vi "Keithley 24XX Output List and Acquire.vi"() -> ()   [LabVIEW 2022 SP3]
doc: "Outputs a sequence of voltages based on a list and takes readings at each point."
uses:
  Keithley 24XX.lvlib
  Initialize Folder/D/Download/Keithley 24XX/Public/Data/Read (Multiple Points).vi
panel:
  in  "Source Mode  (0: Voltage)":u16(ring) items=["Voltage", "Current"]
  in  "Output List":dbl[](array[numeric])=[0.1, 0.2, 0.3]
  in  "VISA resource name":refnum<visa-resource-name>
  in  "Serial Configuration":T1={"Baud Rate"=9600, "Parity"=0, "Data Bits"=8, "Stop Bits"=10, "Flow Control"=0} {"Flow Control" items=["None", "XON/XOFF", "RTS/CTS", "XON/XOFF & RTS/CTS", "DTR/DSR", "XON/XOFF & DTR/DSR"]; "Stop Bits" items=["1.0"=10, "1.5"=15, "2.0"=20]; "Data Bits" items=["7"=7, "8"=8]; "Parity" items=["None", "Odd", "Even", "Mark", "Space"]; "Baud Rate" items=["300"=300, "600"=600, "1200"=1200, "2400"=2400, "4800"=4800, "9600"=9600, "19200"=19200]}
  out "Waveform Graph":sgl[][](graph)
  in  "Timeout (10000 ms)":i32=10000 format="%#.6g"
  in  "Compliance  Level (0.1)":dbl=0.1
  # "(c) 2006 - 2015 National Instruments.  ALL RIGHTS RESERVED."
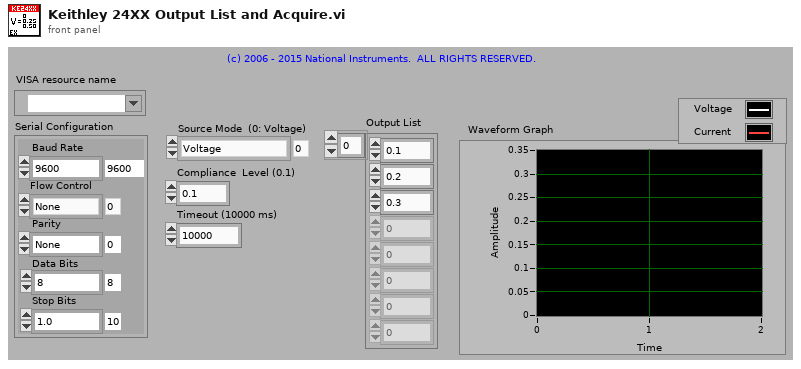
[diagram p1: front panel]
types:
  T1 = cluster{"Baud Rate":u32, "Parity":u16, "Data Bits":u16, "Stop Bits":u16, "Flow Control":u16}
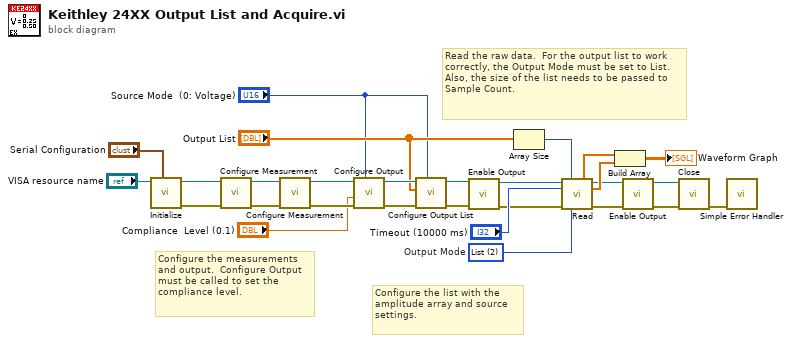
[diagram p0: block diagram]
diagram:
  w17 = u16 2 items=["Fixed", "Sweep", "List"]  # Output Mode
  # "Read the raw data.  For the output list to work correctly, the Output Mode must be set to List.  Also, the size of the list needs to be passed to Sample Count."
  # "Configure the list with the amplitude array and source settings."
  # "Configure the measurements and output.  Configure Output must be called to set the compliance level."
  n1 = call "Initialize.vi"("Serial Configuration"="Serial Configuration", "VISA resource name"="VISA resource name") -> ("error out"=w27:errorcluster, "VISA resource name out"=w28:refnum<visa-resource-name>)  [unwired: 8 in]
  n2 = call "Configure Measurement.vi"("error in (no error)"=w27, "VISA resource name"=w28) -> ("error out"=w26:errorcluster, "VISA resource name out"=w25:refnum<visa-resource-name>)  [unwired: 8 in]
  n3 = call "Configure Measurement.vi"("error in (no error)"=w26, "VISA resource name"=w25) -> ("error out"=w23:errorcluster, "VISA resource name out"=w24:refnum<visa-resource-name>)  [unwired: 8 in]
  n4 = call "Configure Output.vi"("Source Mode  (0: Voltage)"="Source Mode  (0: Voltage)", "error in (no error)"=w23, "Compliance  Level (0.1)"="Compliance  Level (0.1)", "VISA resource name"=w24) -> ("error out"=w19:errorcluster, "VISA resource name out"=w20:refnum<visa-resource-name>)  [unwired: 6 in]
  n5 = call "Configure Output List.vi"("Source Mode  (0: Voltage)"="Source Mode  (0: Voltage)", "error in (no error)"=w19, "Output List"="Output List", "VISA resource name"=w20) -> ("error out"=w9:errorcluster, "VISA resource name out"=w10:refnum<visa-resource-name>)  [unwired: 6 in]
  n6 = call "Enable Output.vi"("error in (no error)"=w9, "VISA resource name"=w10) -> ("error out"=w7:errorcluster, "VISA resource name out"=w8:refnum<visa-resource-name>)  [unwired: 8 in]
  n7 = Array Size(array="Output List") -> (size(s)=w18:i32)
  n8 = call-poly "Read.vi"("VISA resource name"=w8, "Sample Count (1)"=w18, "Timeout (10000 ms)"="Timeout (10000 ms)", "error in (no error)"=w7, "Output Mode (0: Fixed)"=w17) -> ("Voltage"=w15:sgl[], "VISA resource name out"=w4:refnum<visa-resource-name>, "Current"=w14:sgl[], "error out"=w3:errorcluster)  [unwired: 4 in, 3 out]
  n9 = Build Array(w15, w14) -> (→"Waveform Graph":sgl[][])
  n10 = call "Enable Output.vi"("error in (no error)"=w3, "VISA resource name"=w4) -> ("error out"=w6:errorcluster, "VISA resource name out"=w5:refnum<visa-resource-name>)  [unwired: 8 in]
  n11 = call "Close.vi"("error in (no error)"=w6, "VISA resource name"=w5) -> ("error out"=w12:errorcluster)  [unwired: 9 in]
  n12 = call <vilib>:"Simple Error Handler.vi"("error in (no error)"=w12) -> ()  [unwired: 4 in, 5 out]
